vi "Write_Wrap_Simple.vi"(4 "Value":T1) -> (1 "Var":refnum<class "Var_I32.lvclass">)   [LabVIEW 2021, in "Var_I32.lvclass"]
uses:
  Var_I32.lvclass
  Type.ctl
  Var_I32.lvclass/Var_I32.ctl
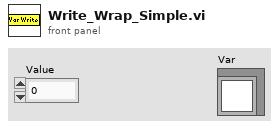
[diagram p1: front panel]
types:
  T1 = typedef "Var_I32.lvclass/Type.ctl" = dbl
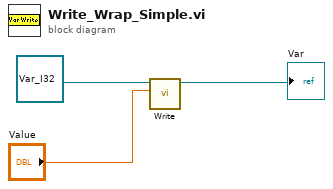
[diagram p0: block diagram]
diagram:
  n1 = call-dynamic "Write.vi"("Value"="Value", "Double Float.lvclass_340760 in"=refnum<class "Var_I32.lvclass"> refnum ("Constants.lvlib:Numeric.lvclass")) -> ("Double Float.lvclass_340760 out"=→"Var":refnum<class "Var_I32.lvclass">)  [unwired: 8 in, 1 out]
